vi "ULS Mover.vi"   [LabVIEW 2016]
uses:
  Class/IFD/IFD.lvclass
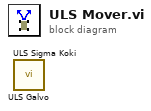
[diagram p0: block diagram]
diagram:
  n1 = call "ULS Galvo.vi"() -> ()  [unwired: 10 in, 2 out]
  n2 = call "ULS Sigma Koki.vi"() -> ()  [unwired: 10 in, 2 out]
